vi "omicron-pressure-logger.vi"() -> ()   [LabVIEW 2016]
uses:
  <vilib>/addons/h5labview2/file/H5Fmode.ctl
  <vilib>/NI/Modbus Library/API/Wrapper/Create Serial Master.vi
  <vilib>/NI/Modbus Library/API/Master/Modbus Master.lvclass
  <vilib>/NI/Modbus Library/API/Wrapper/API Main.lvlib
  <vilib>/addons/h5labview2/file/H5F.lvlib
  <vilib>/addons/h5labview2/dataset/H5D.lvlib
panel:
  out "Waveform Chart":waveform(sgl)[](graph)
  out "lt":sgl format="%_3e"
  in  "quit":bool
  out "oil pump  (mbar)":sgl format="%#.3g"
  out "prep":sgl caption="PREP" format="%_3e"
  # "mbar"
  # "mbar"
  # "prep"
  # "lt"
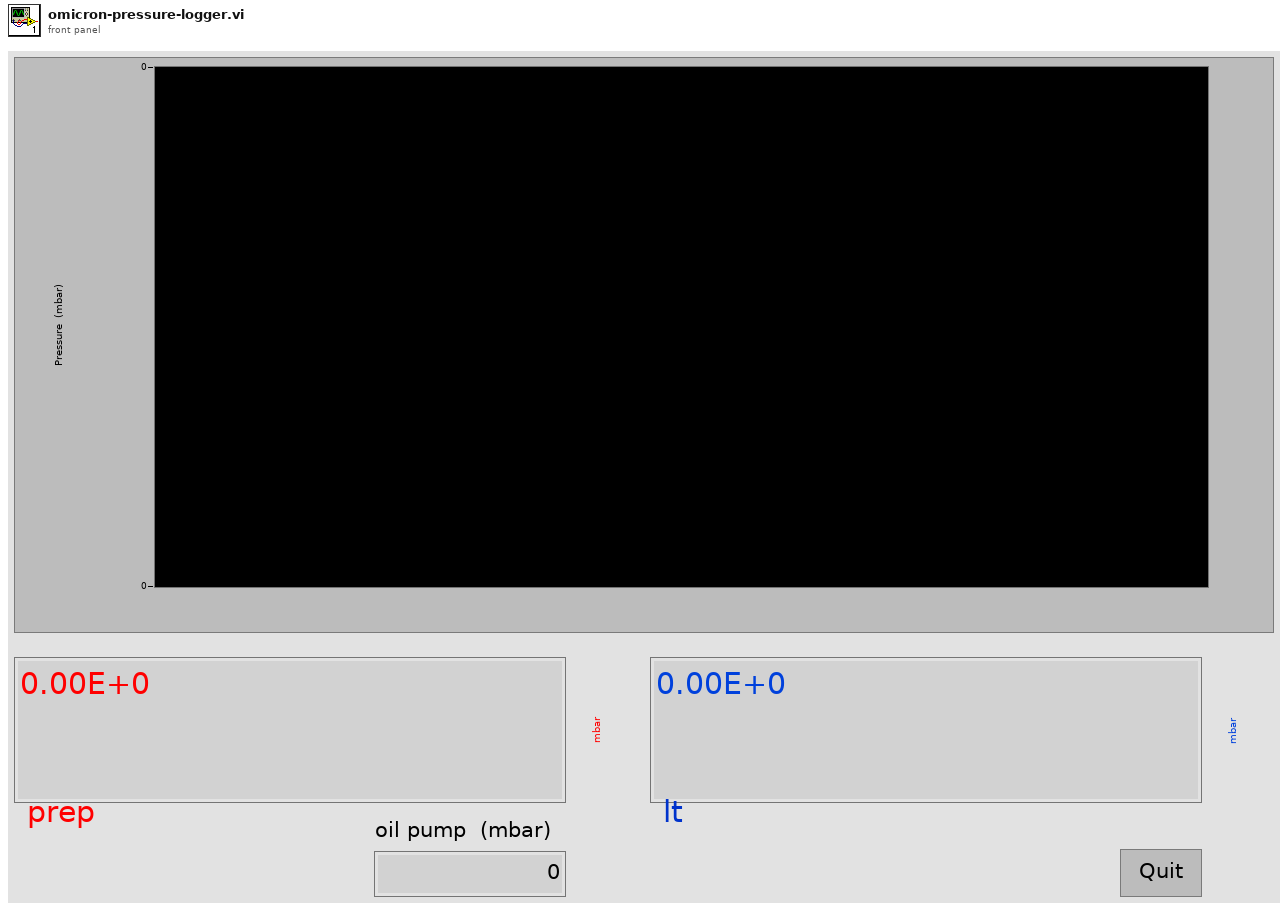
[diagram p1: front panel]
types:
  T1 = typedef "H5F.lvlib/H5Fmode.ctl" = enum16{"read-only", "read-write", "overwrite", "create new", "open or create"}
  T2 = enum16{"open", "replace", "create", "open or create", "replace or create", "replace or create with confirmation"}
  T3 = typedef "hid_t.ctl" = i32
  T4 = cluster{"timestamp":timestamp, "time <19>":string, "prep":sgl, "lt":sgl, "oil pump":sgl}
  T5 = cluster{"timestamp":timestamp, "time <19>":string, "prep":sgl, "lt":sgl, "oil pump":sgl}[]
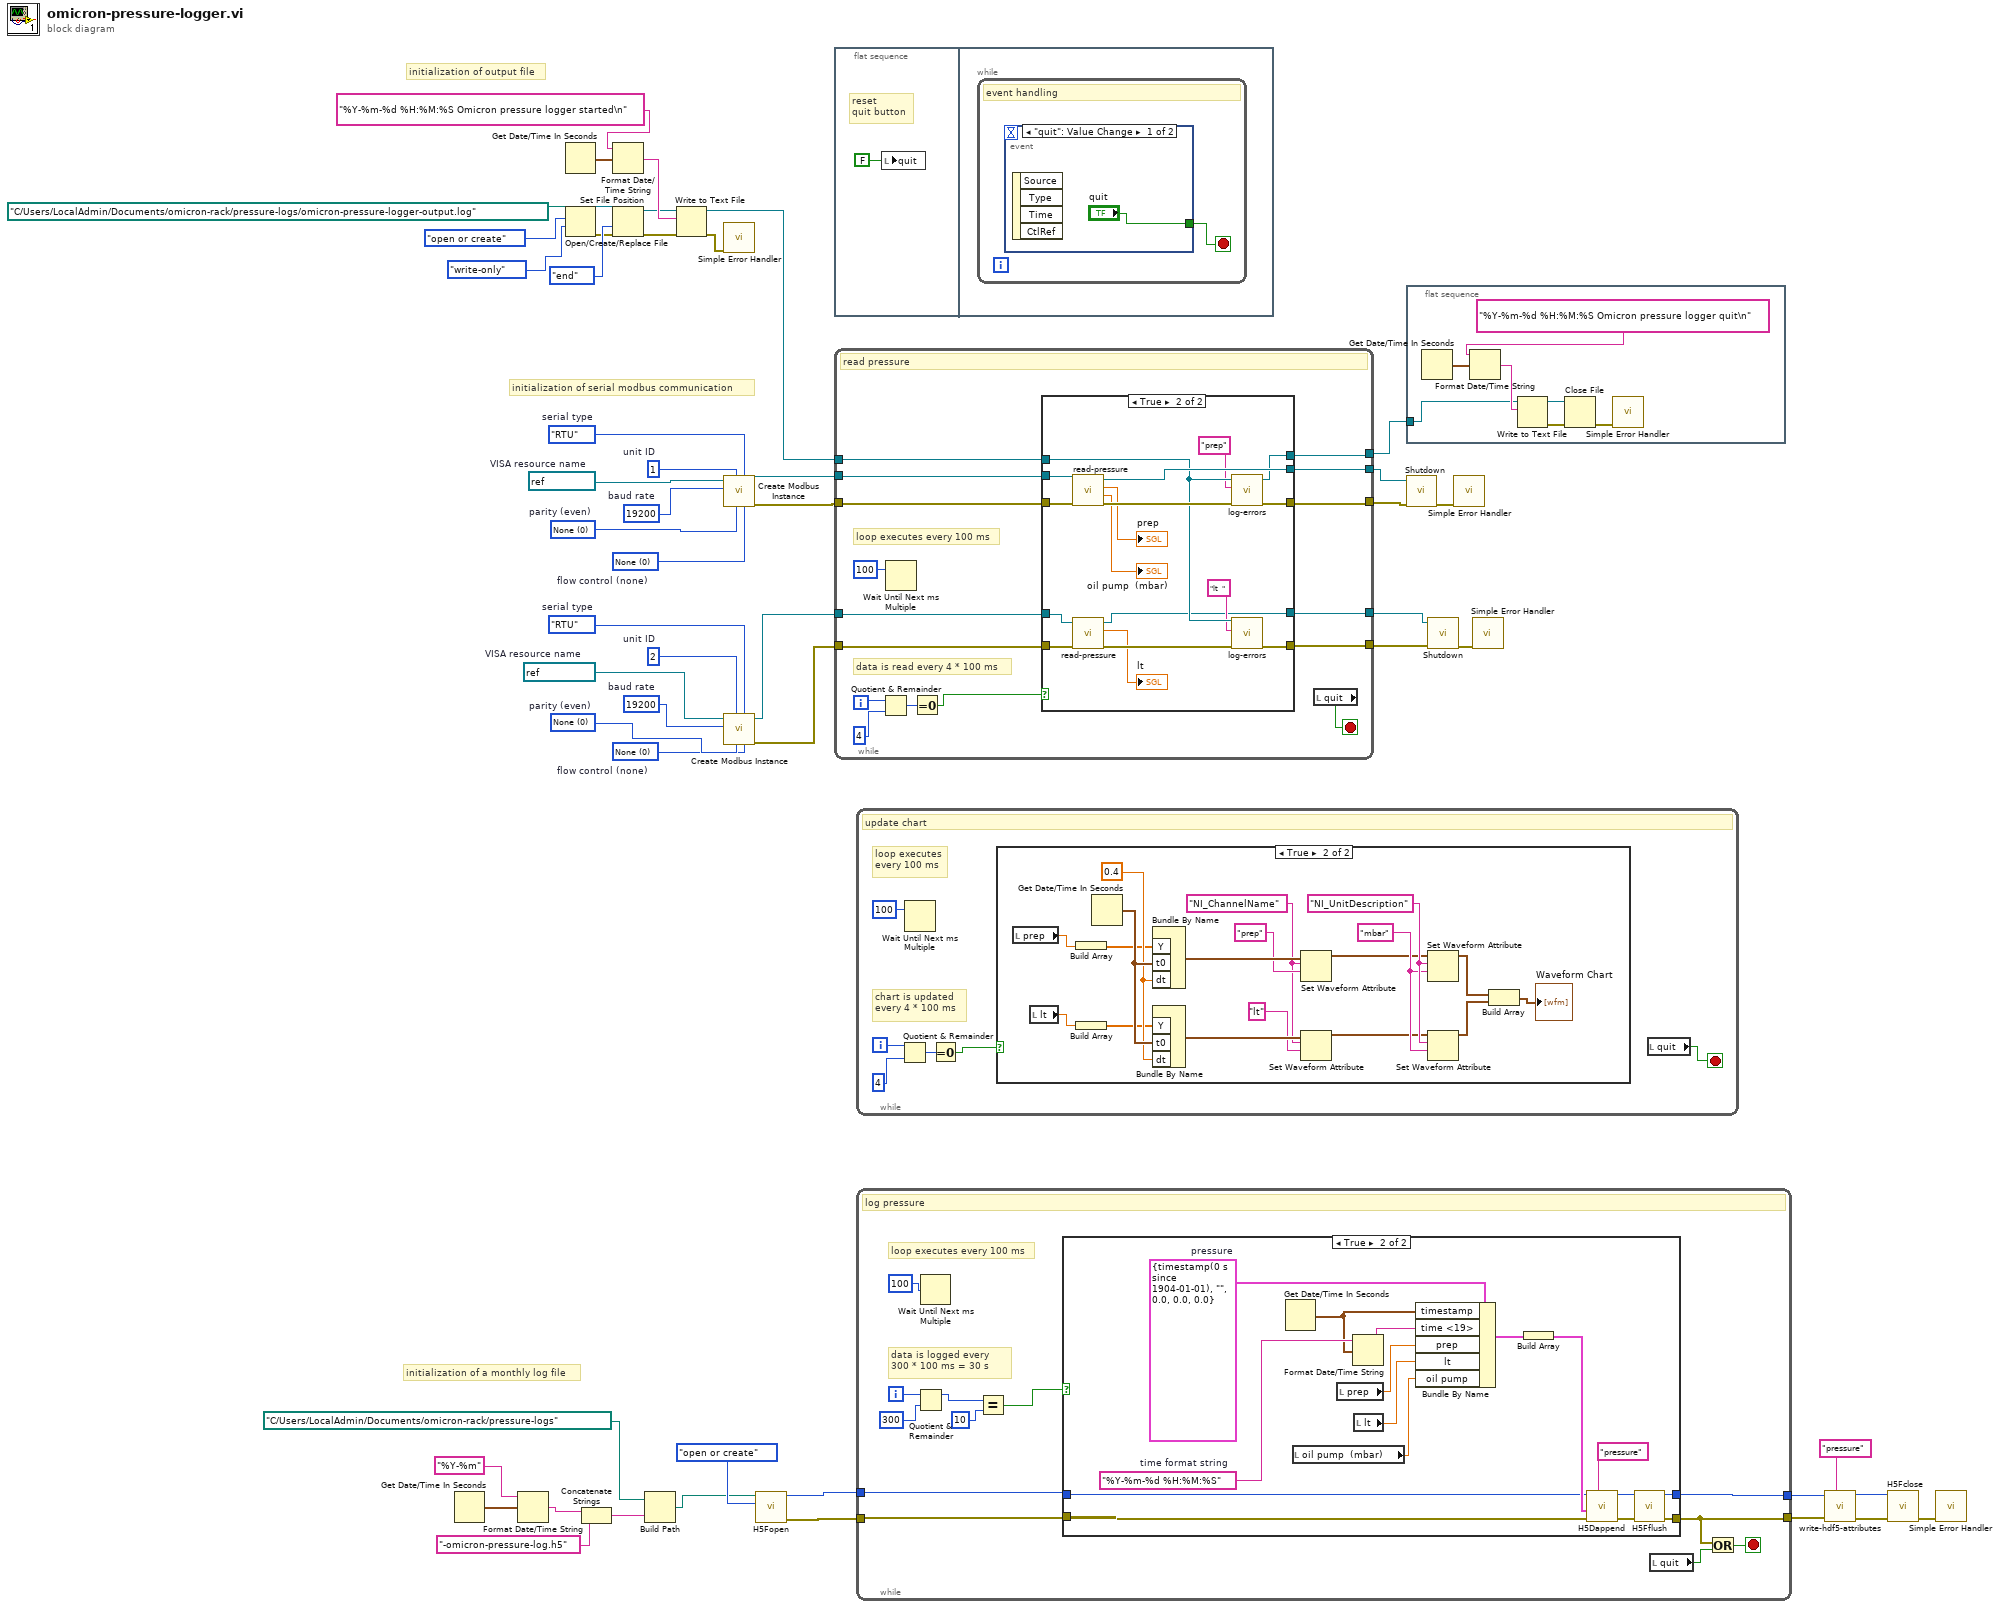
[diagram p0: block diagram]
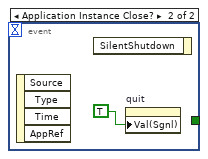
[diagram p3: hidden frame]
diagram:
  w31 = u16 0 items=["None", "XON/XOFF", "RTS/CTS", "XON/XOFF & RTS/CTS", "DTR/DSR", "XON/XOFF & DTR/DSR"]  # flow control (none)
  w32 = u16 0 items=["None", "Odd", "Even", "Mark", "Space"]  # parity (even)
  w35 = u32 19200  # baud rate
  w36 = refnum<visa-resource-name> "COM12"  # VISA resource name
  w34 = u8 2  # unit ID
  w33 = enum16{"RTU", "ASCII"}."RTU"  # serial type
  w43 = u16 0 items=["None", "XON/XOFF", "RTS/CTS", "XON/XOFF & RTS/CTS", "DTR/DSR", "XON/XOFF & DTR/DSR"]  # flow control (none)
  w44 = u16 0 items=["None", "Odd", "Even", "Mark", "Space"]  # parity (even)
  w47 = u32 19200  # baud rate
  w48 = refnum<visa-resource-name> "COM11"  # VISA resource name
  w46 = u8 1  # unit ID
  w45 = enum16{"RTU", "ASCII"}."RTU"  # serial type
  # "initialization of serial modbus communication"
  # "initialization of a monthly log file"
  # "initialization of output file"
  n1 = Get Date/Time In Seconds() -> (seconds since 1Jan1904=w28:timestamp)
  n2 = Format Date/Time String(time format string (%c)="%Y-%m", seconds (now)=w28) -> (date/time string=w26:string)  [unwired: 1 in]
  n3 = Get Date/Time In Seconds() -> (seconds since 1Jan1904=w9:timestamp)
  n4 = Open/Create/Replace File(file path (use dialog)=path "C:/Users/LocalAdmin/Documents/omicron-rack/pressure-logs/omicron-pressure-logger-output.log" ("Path"), operation (0:open)=T2."open or create", access (0:read/write)=enum16{"read/write", "read-only", "write-only"}."write-only") -> (refnum out=w40:refnum<file>, error out=w4:errorcluster)  [unwired: 3 in, 1 out]
  n5 = Concatenate Strings(w26, "-omicron-pressure-log.h5" ("string")) -> (w23:string)
  n6 = Format Date/Time String(time format string (%c)="%Y-%m-%d %H:%M:%S Omicron pressure logger started\n", seconds (now)=w9) -> (date/time string=w8:string)  [unwired: 1 in]
  n7 = Set File Position(refnum=w40, from (0:start)=enum16{"start", "end", "current"}."end", error in=w4) -> (refnum out=w6:refnum<file>, error out=w3:errorcluster)  [unwired: 1 in]
  n8 = Build Path(base path=path "C:/Users/LocalAdmin/Documents/omicron-rack/pressure-logs" ("path"), name or relative path=w23) -> (appended path=w11:path)
  n9 = Write to Text File(file (use dialog)=w6, text=w8, error in=w3) -> (refnum out=w5:refnum<file>, error out=w2:errorcluster)  [unwired: 1 in, 1 out]
  n10 = call <vilib>:"Simple Error Handler.vi"("error in (no error)"=w2) -> ()  [unwired: 4 in, 5 out]
  n11 = call-poly <vilib>:"Create Modbus Instance.vi"("flow control (none)"=w43, "serial type"=w45, "parity (even)"=w44, "unit ID"=w46, "baud rate"=w47, "VISA resource name"=w48) -> ("error out"=w51:errorcluster, "serial master instance"=w52:refnum<class "Modbus Master.lvclass">)  [unwired: 4 in]
  n12 = call-poly <vilib>:"Create Modbus Instance.vi"("flow control (none)"=w31, "serial type"=w33, "parity (even)"=w32, "unit ID"=w34, "baud rate"=w35, "VISA resource name"=w36) -> ("error out"=w29:errorcluster, "serial master instance"=w30:refnum<class "Modbus Master.lvclass">)  [unwired: 4 in]
  n13 = call <vilib>:"H5Fopen.vi"("mode (read-only)"=H5Fmode."open or create", "path"=w11) -> ("error out"=w21:errorcluster, "ref out"=w22:T3)  [unwired: 8 in]
  n14 = flat-sequence {
    frame #0 {
      # "reset\nquit button"
      n15 = local write "quit"(FALSE) -> ()
    }
    frame #1 {
      n16 = while {
        stop <- w54 stop-if-true
        # "event handling"
        n17 = event shown="[0] \"quit\": Value Change" {
          selector: _ -> [_ _]
          dyn-events: _ -> [_ _]
          timeout: _ -> [_ _]
          tunnel: ["quit" _] -> w54
          event "quit": Value Change {
            n18 = event-data() -> ()  [unwired: 1 in, 4 out]
          }
          event Application Instance Close? {
            n19 = event-data() -> ()  [unwired: 1 in, 4 out]
            n20 = event-data() -> ()  [unwired: 2 in, 1 out]
            n21 = property on="quit" class="Bool (strict)"("Val(Sgnl)"=TRUE) -> ()  [unwired: 2 in, 2 out]
          }
        }
      }
    }
  }
  n22 = while {
    tunnel: w30 -> [w60]
    tunnel: w29 -> [w59]
    tunnel: [w58] -> w19
    tunnel: w51 -> [w64]
    tunnel: [w61] -> w49
    tunnel: w52 -> [w65]
    tunnel: [w62] -> w50
    tunnel: w5 -> [w66]
    tunnel: [w63] -> w1
    tunnel: [w57] -> w20
    i -> [w67]
    stop <- w72 stop-if-true
    # "data is read every 4 * 100 ms"
    # "loop executes every 100 ms"
    # "read pressure"
    n23 = Quotient & Remainder(x=w67, y=4) -> (x-y*floor(x/y)=w69:i32)  [unwired: 1 out]
    n24 = Wait Until Next ms Multiple(millisecond multiple=u32 100 ("milliseconds to wait")) -> ()  [unwired: 1 out]
    n25 = Equal To 0?(x=w69) -> (x = 0?=w68:bool)
    n26 = case shown="True" w68 {
      tunnel: w66 -> [w77 w83]
      tunnel: w65 -> [w75 w92]
      tunnel: w64 -> [w76 w91]
      tunnel: [w77 w87] -> w63
      tunnel: [w76 w88] -> w61
      tunnel: [w75 w89] -> w62
      tunnel: w60 -> [w73 w86]
      tunnel: w59 -> [w74 w85]
      tunnel: [w74 w84] -> w58
      tunnel: [w73 w78] -> w57
      frame False {
      }
      frame True {
        n27 = call "read-pressure.vi"("error in"=w91, "Modbus instance in"=w92) -> ("error out"=w94:errorcluster, "Pirani"=→"oil pump  (mbar)":sgl, "Ion Gauge"=→"prep":sgl, "Modbus instance out"=w89:refnum<class "Modbus Master.lvclass">)  [unwired: 6 in]
        n28 = call "read-pressure.vi"("error in"=w85, "Modbus instance in"=w86) -> ("error out"=w90:errorcluster, "Ion Gauge"=→"lt":sgl, "Modbus instance out"=w78:refnum<class "Modbus Master.lvclass">)  [unwired: 6 in, 1 out]
        n29 = call "log-errors.vi"("error in (no error)"=w94, "device"="prep", "refnum in"=w83) -> ("error out"=w88:errorcluster, "refnum out"=w87:refnum<file>)  [unwired: 7 in]
        n30 = call "log-errors.vi"("error in (no error)"=w90, "device"="lt  ", "refnum in"=w83) -> ("error out"=w84:errorcluster)  [unwired: 7 in, 1 out]
      }
    }
    n31 = local read "quit"() -> (w72:bool)
  }
  n32 = while {
    i -> [w96]
    stop <- w95 stop-if-true
    # "chart is updated\nevery 4 * 100 ms"
    # "loop executes\nevery 100 ms"
    # "update chart"
    n33 = Quotient & Remainder(x=w96, y=4) -> (x-y*floor(x/y)=w98:i32)  [unwired: 1 out]
    n34 = Wait Until Next ms Multiple(millisecond multiple=u32 100 ("milliseconds to wait")) -> ()  [unwired: 1 out]
    n35 = Equal To 0?(x=w98) -> (x = 0?=w97:bool)
    n36 = case shown="True" w97 {
      frame False {
      }
      frame True {
        w105 = "mbar" ("name")
        w106 = "NI_UnitDescription" ("name")
        w112 = "NI_ChannelName" ("name")
        w117 = 0.4 ("dt")
        n37 = local read "prep"() -> (w110:sgl)
        n38 = local read "lt"() -> (w108:sgl)
        n39 = Build Array(w110) -> (w109:sgl[])
        n40 = Build Array(w108) -> (w107:sgl[])
        n41 = Get Date/Time In Seconds() -> (seconds since 1Jan1904=w118:timestamp)
        n42 = Bundle By Name("Y"=w109, "t0"=w118, "dt"=w117) -> (w115:waveform(sgl))  [unwired: 1 in]
        n43 = Bundle By Name("Y"=w107, "t0"=w118, "dt"=w117) -> (w113:waveform(sgl))  [unwired: 1 in]
        n44 = Set Waveform Attribute(5:"prep" ("name"), 6:w112, 7:w115) -> (3:w104:waveform(sgl))  [unwired: 1 in, 2 out]
        n45 = Set Waveform Attribute(5:"lt" ("name"), 6:w112, 7:w113) -> (3:w103:waveform(sgl))  [unwired: 1 in, 2 out]
        n46 = Set Waveform Attribute(5:w105, 6:w106, 7:w104) -> (3:w102:waveform(sgl))  [unwired: 1 in, 2 out]
        n47 = Set Waveform Attribute(5:w105, 6:w106, 7:w103) -> (3:w101:waveform(sgl))  [unwired: 1 in, 2 out]
        n48 = Build Array(w102, w101) -> (→"Waveform Chart":waveform(sgl)[])
      }
    }
    n49 = local read "quit"() -> (w95:bool)
  }
  n50 = while {
    tunnel: w22 -> [w125]
    tunnel: [w123] -> w17
    tunnel: w21 -> [w124]
    tunnel: [w122] -> w16
    i -> [w127]
    stop <- w119 stop-if-true
    # "data is logged every\n300 * 100 ms = 30 s"
    # "loop executes every 100 ms"
    # "log pressure"
    n51 = Quotient & Remainder(x=w127, y=300) -> (x-y*floor(x/y)=w121:i32)  [unwired: 1 out]
    n52 = Wait Until Next ms Multiple(millisecond multiple=u32 100 ("milliseconds to wait")) -> ()  [unwired: 1 out]
    n53 = Equal?(x=w121, y=10) -> (x = y?=w126:bool)
    n54 = case shown="True" w126 {
      tunnel: w125 -> [w132 w144]
      tunnel: w124 -> [w131 w143]
      tunnel: [w132 w139] -> w123
      tunnel: [w131 w141] -> w122
      frame False {
      }
      frame True {
        w138 = "%Y-%m-%d %H:%M:%S"  # time format string
        w148 = T4 {"timestamp"=timestamp(0 s since 1904-01-01), "time <19>"="", "prep"=0.0, "lt"=0.0, "oil pump"=0.0}  # pressure
        n55 = Get Date/Time In Seconds() -> (seconds since 1Jan1904=w137:timestamp)
        n56 = local read "oil pump  (mbar)"() -> (w133:sgl)
        n57 = local read "prep"() -> (w135:sgl)
        n58 = Format Date/Time String(time format string (%c)=w138, seconds (now)=w137) -> (date/time string=w136:string)  [unwired: 1 in]
        n59 = local read "lt"() -> (w134:sgl)
        n60 = Bundle By Name(cluster=w148, "timestamp"=w137, "time <19>"=w136, "prep"=w135, "lt"=w134, "oil pump"=w133) -> (w147:T4)
        n61 = Build Array(w147) -> (w145:T5)
        n62 = call <vilib>:"H5Dappend.vi"("dataset name"="pressure" ("name"), "error in (no error)"=w143, "data"=w145, "ref in"=w144) -> ("error out"=w142:errorcluster, "ref out"=w140:T3)  [unwired: 4 in, 2 out]
        n63 = call <vilib>:"H5Fflush.vi"("error in (no error)"=w142, "ref in"=w140) -> ("error out"=w141:errorcluster, "ref out"=w139:T3)  [unwired: 8 in]
      }
    }
    n64 = local read "quit"() -> (w130:bool)
    n65 = Or(x=w122, y=w130) -> (x .or. y?=w119:bool)
  }
  n66 = flat-sequence {
    tunnel: w1 -> [w152]
    frame #0 {
      n67 = Get Date/Time In Seconds() -> (seconds since 1Jan1904=w155:timestamp)
      n68 = Format Date/Time String(time format string (%c)="%Y-%m-%d %H:%M:%S Omicron pressure logger quit\n", seconds (now)=w155) -> (date/time string=w154:string)  [unwired: 1 in]
      n69 = Write to Text File(file (use dialog)=w152, text=w154) -> (refnum out=w151:refnum<file>, error out=w150:errorcluster)  [unwired: 2 in, 1 out]
      n70 = Close File(refnum=w151, error in=w150) -> (error out=w149:errorcluster)  [unwired: 1 out]
      n71 = call <vilib>:"Simple Error Handler.vi"("error in (no error)"=w149) -> ()  [unwired: 4 in, 5 out]
    }
  }
  n72 = call-dynamic "Shutdown.vi"("error in"=w49, "Modbus master in"=w50) -> ("error out"=w37:errorcluster)  [unwired: 9 in]
  n73 = call-dynamic "Shutdown.vi"("error in"=w19, "Modbus master in"=w20) -> ("error out"=w18:errorcluster)  [unwired: 9 in]
  n74 = call <vilib>:"Simple Error Handler.vi"("error in (no error)"=w37) -> ()  [unwired: 4 in, 5 out]
  n75 = call <vilib>:"Simple Error Handler.vi"("error in (no error)"=w18) -> ()  [unwired: 4 in, 5 out]
  n76 = call "write-hdf5-attributes.vi"("name"="pressure", "error in (no error)"=w16, "ref in"=w17) -> ("error out"=w14:errorcluster, "ref out"=w15:i32)  [unwired: 7 in]
  n77 = call <vilib>:"H5Fclose.vi"("error in (no error)"=w14, "ref"=w15) -> ("error out"=w38:errorcluster)  [unwired: 9 in]
  n78 = call <vilib>:"Simple Error Handler.vi"("error in (no error)"=w38) -> ()  [unwired: 4 in, 5 out]
